vi "RT Main_Read Cluster.vi"() -> ()   [LabVIEW 2018]
uses:
  TypeDefs/Simple cluster.ctl
  01b3861e-4d80-44b0-aa8e-021a80e4586e.vi
  01b3861e-4d80-44b0-aa8e-021a80e4586e.vi/093606d2-6890-4029-a1f1-75edae9247dc.vi
  FPGA Bitfile Register Operations/Scalar IO Operations/Utilities/Find Register Offset.vi
  FPGA Bitfile Register Operations/Scalar IO Operations/Utilities/Parser Cluster Configuration.vi
  FPGA Bitfile Register Operations/Scalar IO Operations/Read Methods/Read U8 Array.vi
  FPGA Bitfile Register Operations/Scalar IO Operations/Utilities/Convert Cluster BLOB to Bool Array.vi
  FPGA Bitfile Register Operations/Scalar IO Operations/Utilities/FXP to DBL.vi
  <userlib>/_OpenG.lib/lvdata/lvdata.llb/Array of VData to VCluster__ogtk.vi
  <vilib>/FPGAPlugInAG/Dynamic/niLvFpga_Close_Dynamic.vi
  <vilib>/rvi/interface/nirviCloseFPGA/nirviCloseFPGA.xnode
  FPGA Bitfile Register Operations/Scalar IO Operations/Scalar IO Operations.lvlib
panel:
  out "Average seconds per read":dbl
  out "Cluster out":T1
  out "error out":errorcluster
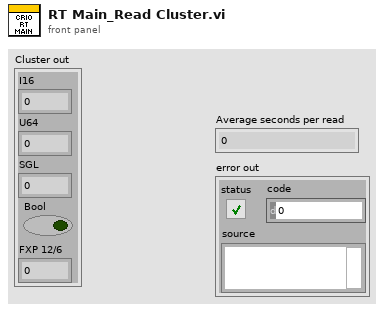
[diagram p1: front panel]
types:
  T1 = typedef "Simple cluster.ctl" = cluster{"I16":i16, "U64":u64, "SGL":sgl, "Bool":bool, "FXP 12/6":fxp<+/-,12,6>}
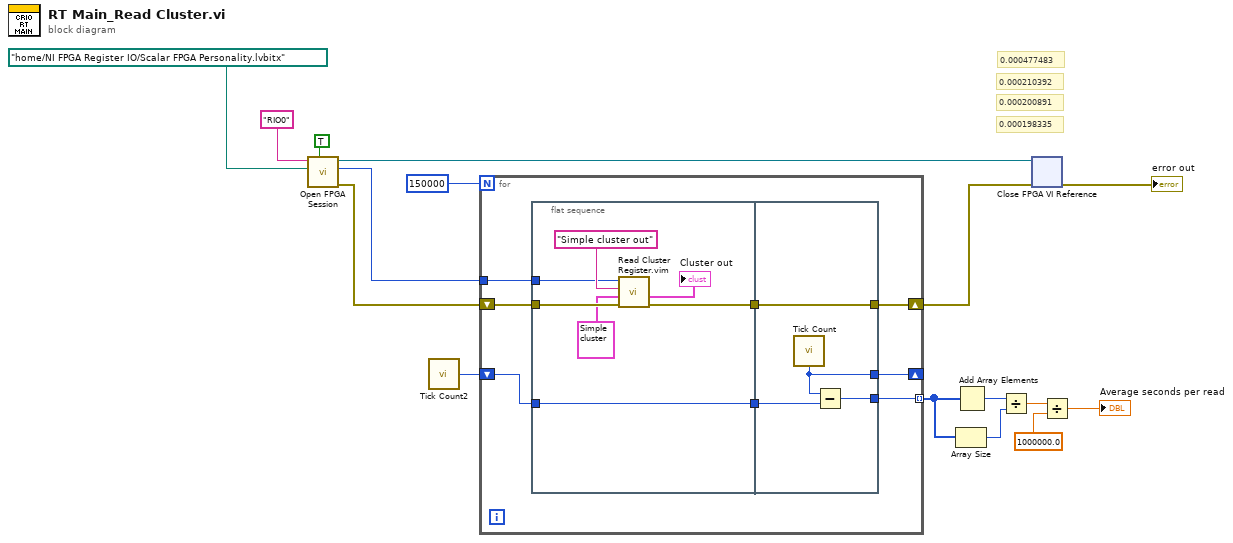
[diagram p0: block diagram]
diagram:
  # "0.000198335"
  # "0.000200891"
  # "0.000210392"
  # "0.000477483"
  n1 = call "Open FPGA Session.vi"("run when loaded (T)"=TRUE ("Run When Loaded (T)"), "bitfile path"=path "/home/NI FPGA Register IO/Scalar FPGA Personality.lvbitx" ("Bitfile path"), "device address"="RIO0" ("Device address")) -> ("error out"=w3:errorcluster, "session out"=w2:u64, "bitfile reference out"=w13:refnum<k20>)  [unwired: 6 in]
  n2 = call "Tick Count2"() -> ("Tick Count(uSec)"=w10:u32)
  n3 = for {
    N: 150000 -> [_]
    shift-right: [w23] -> w1
    shift-left: w3 -> [w24]
    shift-right: [w19] -> _
    shift-left: w10 -> [w21]
    tunnel: [w18] -> w9 mode=indexing
    tunnel: w2 -> [w17]
    n4 = flat-sequence {
      tunnel: w24 -> [w29]
      tunnel: [w28] -> w22
      tunnel: w21 -> [w31]
      tunnel: [w31] -> w20
      tunnel: w17 -> [w27]
      tunnel: [w35] -> w23
      tunnel: w22 -> [w35]
      tunnel: w20 -> [w34]
      tunnel: [w33] -> w19
      tunnel: [w32] -> w18
      frame #0 {
        n5 = call "Read Cluster Register.vim"("error in (no error)"=w29, "Cluster in (default value)"=T1 {"I16"=0, "U64"=0, "SGL"=0.0, "Bool"=FALSE, "FXP 12/6"=0.0} ("Simple Cluster"), "Cluster Name"="Simple cluster out" ("register name"), "session in"=w27) -> ("error out"=w28:errorcluster, "Cluster out"=→"Cluster out":T1)  [unwired: 5 in, 1 out]
      }
      frame #1 {
        n6 = call "Tick Count"() -> ("Tick Count(uSec)"=w33:u32)
        n7 = Subtract(x=w33, y=w34) -> (x-y=w32:u32)
      }
    }
  }
  n8 = Array Size(array=w9) -> (size(s)=w7:i32)
  n9 = Add Array Elements(numeric array=w9) -> (sum=w8:u32)
  n10 = Divide(x=w8, y=w7) -> (x/y=w6:dbl)
  n11 = xnode "Close FPGA VI Reference"("FPGA VI Reference In"=w13, "error in"=w1) -> ("error out"=→"error out":errorcluster)
  n12 = Divide(x=w6, y=1000000.0) -> (x/y=→"Average seconds per read":dbl)
